vi "DSF.Shared.Configuration.Channel.Get Offset.vi"(11 "Channel Configuration in":refnum<class "DSF.Shared.Configuration.Channel Array.lvclass">) -> (2 "buffer offset":u64, 3 "Channel Configuration out":refnum<class "DSF.Shared.Configuration.Channel Array.lvclass">)   [LabVIEW 2016, in "DSF.Shared.lvlib" / "DSF.Shared.Configuration.Channel Array.lvclass"]
uses:
  DSF.Shared.Configuration.Channel Array.lvclass
  DSF.Shared.Configuration.Channel Array.lvclass/DSF.Shared.Configuration.Channel Array.ctl
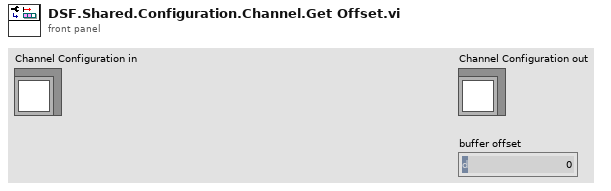
[diagram p1: front panel]
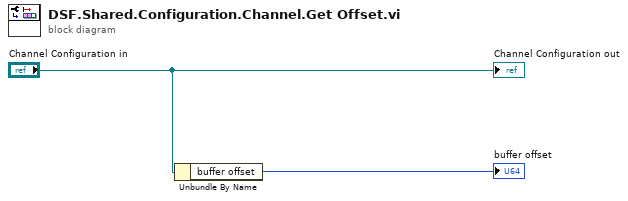
[diagram p0: block diagram]
diagram:
  n1 = Unbundle By Name("Channel Configuration in") -> ("buffer offset"=→"buffer offset":u64)
  "Channel Configuration out" <- "Channel Configuration in"
